vi "Select Key File.vi"(7 "Key Type":T1, 8 "Error In":errorcluster, 11 "Key File In":path) -> (0 "Error Out":errorcluster, 3 "Key File Out":path)   [LabVIEW 2018, in "Tests.lvlib"]
uses:
  Tests.lvlib
  SSH Key Types.ctl
  <vilib>/Utility/sysdir.llb/System Directory Type.ctl
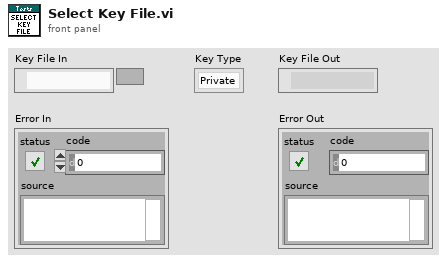
[diagram p1: front panel]
types:
  T1 = typedef "Tests.lvlib/SSH Key Types.ctl" = enum16{"Private", "Public"}
  T2 = typedef "System Directory Type.ctl" = i32
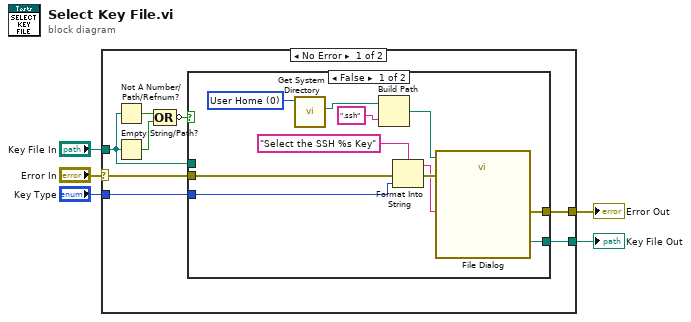
[diagram p0: block diagram]
diagram:
  n1 = case shown="No Error" "Error In" {
    selector: "Error In" -> [w10 w27]
    tunnel: "Key Type" -> [w13 _]
    tunnel: [w12 w27] -> w4
    tunnel: [w11 _] -> w3
    tunnel: "Key File In" -> [w7 _]
    frame No Error {
      n2 = Not A Number/Path/Refnum?(number/path/refnum=w7) -> (NaN/Path/Refnum?=w8:bool)
      n3 = Empty String/Path?(string/path=w7) -> (empty?=w9:bool)
      n4 = Compound Arithmetic op=OR(w8, w9) -> (invert w6:bool)
      n5 = case shown="False" w6 {
        tunnel: w10 -> [w24 w25]
        tunnel: [w23 w25] -> w12
        tunnel: [w22 w26] -> w11
        tunnel: w7 -> [_ w26]
        tunnel: w13 -> [w16 _]
        frame False {
          w21 = T2 0 items=["User Home"=0, "User Desktop"=1, "User Documents"=2, "User Application Data"=3, "User Preferences"=4, "User Temporary"=5, "Public Documents"=6, "Public Application Data"=7, "Public Preferences"=8, "Public Cache"=13, "System Core Libraries"=9, "System Installed Libraries"=10, "Application Files"=11, "Boot Volume Root"=12] ("system directory type")
          n6 = call <vilib>:"Get System Directory.vi"("system directory type"=w21) -> ("system directory"=w20:path)  [unwired: 10 in]
          n7 = Build Path(base path=w20, name or relative path=".ssh") -> (appended path=w18:path)
          n8 = Format Into String(format string="Select the SSH %s Key", error in=w24, w16) -> (resulting string=w14:string, error out=w17:errorcluster)  [unwired: 1 in]
          n9 = call "File Dialog"("start path"=w18, "prompt"=w14, "error in"=w17) -> ("selected path"=w22:path, "error out"=w23:errorcluster)  [unwired: 9 in, 2 out]
        }
        frame True {
        }
      }
    }
    frame Error {
    }
  }
  "Error Out" <- w4
  "Key File Out" <- w3
